vi "acq.constructImage.vi"(7 "DVR":T1, 8 "error in":errorcluster, 9 "queue2 in":refnum<queue>, 10 "queue1 in":refnum<queue>) -> (0 "error out":errorcluster, 1 "Dark":u16[][](array[numeric]), 2 "PL":u16[][](array[numeric]), 3 "Bright":u16[][](array[numeric]))   [LabVIEW 2020]
uses:
  _controls/data.ref.ctl
  _controls/state.ctl
  _controls/data.vars.ctl
  _controls/data.ctl
  _controls/flip.ctl
  <vilib>/vision/Image Controls.llb/IMAQ Image.ctl
  camera/camera.lvclass
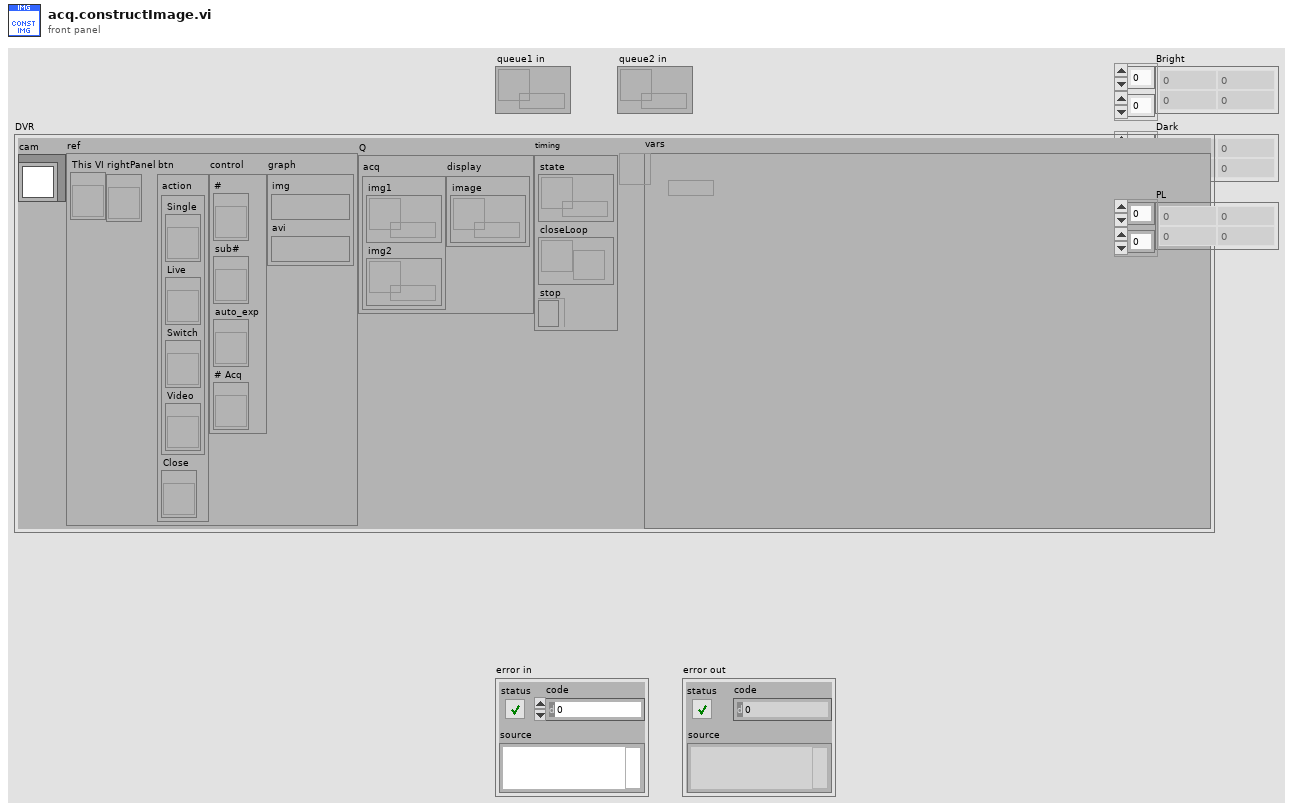
[diagram p1: front panel]
types:
  T1 = typedef "data.ctl" = cluster{"cam":refnum<class "camera.lvclass">, "ref":T2, "Q":cluster{"acq":cluster{"img1":refnum<queue>, "img2":refnum<queue>}, "display":cluster{"image":refnum<queue>}}, "timing":cluster{"state":refnum<queue>, "closeLoop":refnum<notifier>, "stop":refnum<k4>}, "vars":refnum<data-value>}
  T2 = typedef "data.ref.ctl" = cluster{"This VI":refnum<vi>, "rightPanel":refnum<vi>, "btn":cluster{"action":cluster{"Single":refnum<vi>, "Live":refnum<vi>, "Switch":refnum<vi>, "Video":refnum<vi>}, "Close":refnum<vi>}, "control":cluster{"#":refnum<vi>, "sub#":refnum<vi>, "auto_exp":refnum<vi>, "# Acq":refnum<vi>}, "graph":cluster{"img":T3, "avi":T3}}
  T3 = typedef "IMAQ Image.ctl" = refnum<image>
  T4 = typedef "data.vars.ctl" = cluster{"save":cluster{"base_folder":cluster{"Folder":path, "tif":bool, "jpg":bool}, "module":string, "#":u32, "sub#":u8, "save.op":enum16{"Full", "Light"}, "same?":bool, "Shift":enum16{"Single", "Leapfrog"}, "jpg?":bool, "flip":T5}, "acq":cluster{"# Acq":u16, "rotate":bool, "FPS":dbl}, "calib.manual":cluster{"BG":cluster{"Image":u16[][], "enabled?":bool}, "FF":cluster{"Image":u16[][], "enabled?":bool}}}
  T5 = typedef "flip.ctl" = cluster{"x":bool, "y":bool}
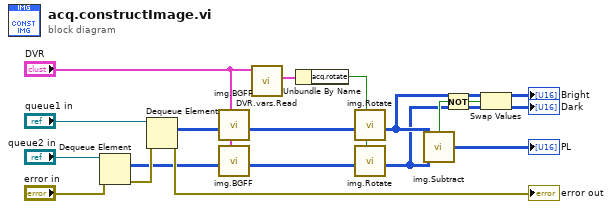
[diagram p0: block diagram]
diagram:
  n1 = Dequeue Element(queue="queue2 in", error in (no error)="error in") -> (element=w7:u16[][], error out=w16:errorcluster)  [unwired: 1 in, 2 out]
  n2 = Dequeue Element(queue="queue1 in", error in (no error)=w16) -> (element=w8:u16[][], error out=→"error out":errorcluster)  [unwired: 1 in, 2 out]
  n3 = call "img.BGFF.vi"("DVR"="DVR", "image in"=w8) -> ("image out"=w4:u16[][])  [unwired: 9 in]
  n4 = call "img.BGFF.vi"("DVR"="DVR", "image in"=w7) -> ("image out"=w3:u16[][])  [unwired: 9 in]
  n5 = call "DVR.vars.Read.vi"("DVR.state"="DVR") -> ("vars"=w6:T4)  [unwired: 9 in, 1 out]
  n6 = Unbundle By Name(w6) -> ("acq.rotate"=w1:bool)
  n7 = call "img.Rotate.vi"("rotate"=w1, "image in"=w4) -> ()  [unwired: 9 in, 1 out]
  n8 = call "img.Rotate.vi"("rotate"=w1, "image in"=w3) -> ("image out"=w2:u16[][])  [unwired: 9 in]
  n9 = call "img.Subtract.vi"("image2 in"=w2, "image1 in"=w4) -> ("Array"=→"PL":u16[][], "x > y?"=w12:bool)
  n10 = Not(x=w12) -> (.not. x?=w9:bool)
  n11 = Swap Values(12:w4, 13:w9, 14:w2) -> (1:→"Bright":u16[][], 3:→"Dark":u16[][])
